vi "Constants.vi"() -> ()   [LabVIEW 2019, in "MD4Logger Shared.lvlib"]
doc: "Use this Global VI to access the GUIDs assigned to the page resources of the Custom Device."
uses:
  MD4Logger Shared.lvlib
panel:
  in  "Tab Control":enum32{"GUIDS", "Constants", "Properties"}(tab)=enum."Constants"
  in  "Commands Folder GUID":string="942972c8-72db-43fa-bc4c-7da23ff4c24d"
  in  "File Name GUID":string="c30a3cba-9920-442c-9814-e12b4247b624"
  in  "MD4Logger GUID":string="1a3b2b0d-9cf3-4849-bac1-3a09abcb7558"
  in  "Channels Folder GUID":string="2a3b2b0d-9cf3-4849-bac1-3a09abcb7558"
  in  "Folder Path GUID":string="3a3b2b0d-9cf3-4849-bac1-3a09abcb7558"
  in  "CommandsFolderName":string="Commands"
  in  "ChannelsFolderName":string="Channels"
  in  "Compiled.Settings":string="Compiled.Settings"
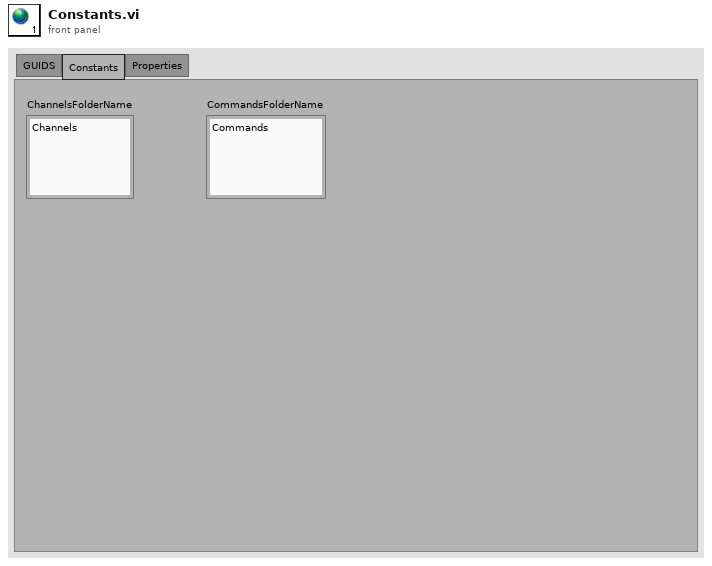
[diagram p1: front panel]
diagram:
